vi "UHR-Fleezers Control (host) - 10.9.vi"() -> ()   [LabVIEW 2011] (continued)
        n1723 = local write "Set Reading to\nSetpoint"(FALSE ("Set SP to Reading")) -> ()
        n1724 = xnode "Read/Write Control"("FPGA VI Reference In"=w2622, "error in"=w2621) -> ("FPGA VI Reference Out"=w2620:T19, "error out"=w2619:errorcluster, "Trap Pos FB Int-Norm Signal"=w2618:fxp<+/-,16,1>)
        n1725 = local read "Differential FB?"() -> (w2623:bool)
        n1726 = case shown="False" w2623 {
          tunnel: [w2628 w2635] -> w2625
          tunnel: w2618 -> [w2626 w2635]
          frame False {
            n1727 = local read "Trap Pos FB Monitor\nT1 or T2"() -> (w2631:bool)
            n1728 = local read "Trap X AI1 (DMA)"() -> (w2634:T13)
            n1729 = Unbundle By Name(w2634) -> ("Set 1"=w2633:fxp<+/-,16,1>, "Set 2"=w2632:fxp<+/-,16,1>)
            n1730 = Select(t=w2633, s=w2631, f=w2632) -> (s? t:f=w2630:fxp<+/-,16,1>)
            n1731 = Not(x="Set SP Using...") -> (.not. x?=w2627:bool)
            n1732 = Select(t=w2626, s=w2627, f=w2630) -> (s? t:f=w2628:fxp<+/-,16,1>)
          }
          frame True {
          }
        }
        n1733 = xnode "Read/Write Control"("FPGA VI Reference In"=w2620, "error in"=w2619, "Trap Pos. FB SP"=w2625) -> ()  [unwired: 2 out]
        n1734 = local write "Trap Pos FB SP"(w2625) -> ()
      }
      event "Trap Pos. FB Out Scale 2^n": Value Change {
        n1735 = event-data() -> ()  [unwired: 7 out]
        n1736 = Scale By Power Of 2(n="Trap Pos. FB Out Scale 2^n", x=ext 1.0) -> (x*2^n=w2636:ext)
        n1737 = property on="Trap Pos. FB Mult Factor" class="DigNum (strict)"("Val(Sgnl)"=w2636) -> ()  [unwired: 2 in, 2 out]
      }
      event "Trap Pos FB Int Count": Value Change {
        n1738 = event-data() -> ()  [unwired: 7 out]
        n1739 = xnode "Read/Write Control"("FPGA VI Reference In"=w2641, "error in"=w2640, "Trap Pos FB Int Count"="Trap Pos FB Int Count") -> ()  [unwired: 2 out]
      }
    }
    "error out 2" <- w1554
    n1740 = node-c288() -> ()  [unwired: 2 out]
  }
  n1741 = timed-loop "Mouse control: trap position (AOM deflection), set confocal spot from image" {
    tunnel: [w2643] -> w182
    tunnel: w50 -> [w2642]
    timing: w94 -> [_]
    timing-out: [_] -> w93
    stop <- w2643 stop-if-true
    n1742 = node-c288() -> ()  [unwired: 2 out]
    n1743 = event shown="[0] \"Pane\": Mouse Down" {
      selector: _ -> [_ _]
      dyn-events: _ -> [_ _]
      timeout: _ -> [_ _]
      tunnel: w2642 -> [w2646 _]
      event Mouse Down {
        n1744 = event-data() -> ("Time"=w2648:u32, "Coords"=w2647:T7, "Button"=w2649:u16)  [unwired: 6 out]
        n1745 = case shown="1" w2649 {
          tunnel: w2648 -> [_ _ w2752]
          tunnel: w2647 -> [_ w2686 w2750]
          tunnel: w2646 -> [_ _ w2748]
          frame 0, Default {
          }
          frame 1 {
            n1746 = property on="APD 2" class="ImageControl"() -> ("Displayed Image Position"=w2656:cluster{"Left":i32, "Top":i32})  [unwired: 2 in, 2 out]
            n1747 = property on="APD 1" class="ImageControl"() -> ("Displayed Image Position"=w2685:cluster{"Left":i32, "Top":i32})  [unwired: 2 in, 2 out]
            n1748 = property on="Detection Laser X" class="ImageControl"() -> ("Displayed Image Position"=w2682:cluster{"Left":i32, "Top":i32})  [unwired: 2 in, 2 out]
            n1749 = property on="Detection Laser Y" class="ImageControl"() -> ("Displayed Image Position"=w2681:cluster{"Left":i32, "Top":i32})  [unwired: 2 in, 2 out]
            n1750 = property on="APD 2" class="ImageControl"() -> ("Displayed Image Size"=w2655:cluster{"Width":u32, "Height":u32})  [unwired: 2 in, 2 out]
            n1751 = property on="APD 1" class="ImageControl"() -> ("Displayed Image Size"=w2683:cluster{"Width":u32, "Height":u32})  [unwired: 2 in, 2 out]
            n1752 = property on="Detection Laser X" class="ImageControl"() -> ("Displayed Image Size"=w2684:cluster{"Width":u32, "Height":u32})  [unwired: 2 in, 2 out]
            n1753 = property on="Detection Laser Y" class="ImageControl"() -> ("Displayed Image Size"=w2680:cluster{"Width":u32, "Height":u32})  [unwired: 2 in, 2 out]
            n1754 = Unbundle By Name(w2655) -> ("Width"=w2652:u32, "Height"=w2651:u32)
            n1755 = Unbundle By Name(w2656) -> ("Left"=w2654:i32, "Top"=w2653:i32)
            n1756 = Unbundle By Name(w2683) -> ("Width"=w2677:u32, "Height"=w2676:u32)
            n1757 = Unbundle By Name(w2684) -> ("Width"=w2673:u32, "Height"=w2672:u32)
            n1758 = Unbundle By Name(w2680) -> ("Width"=w2669:u32, "Height"=w2668:u32)
            n1759 = Unbundle By Name(w2685) -> ("Left"=w2679:i32, "Top"=w2678:i32)
            n1760 = Unbundle By Name(w2682) -> ("Left"=w2675:i32, "Top"=w2674:i32)
            n1761 = Unbundle By Name(w2681) -> ("Left"=w2671:i32, "Top"=w2670:i32)
            n1762 = Bundle("Left"=w2654, "Top"=w2653, "Width"=w2652, "Height"=w2651) -> (w2650:T29)  [unwired: 1 in]
            n1763 = Bundle("Left"=w2679, "Top"=w2678, "Width"=w2677, "Height"=w2676) -> (w2667:T29)  [unwired: 1 in]
            n1764 = Bundle("Left"=w2675, "Top"=w2674, "Width"=w2673, "Height"=w2672) -> (w2666:T29)  [unwired: 1 in]
            n1765 = Bundle("Left"=w2671, "Top"=w2670, "Width"=w2669, "Height"=w2668) -> (w2665:T29)  [unwired: 1 in]
            n1766 = Build Cluster Array(w2650, w2667, w2666, w2665) -> (w2664:T30)
            n1767 = for {
              tunnel: w2686 -> [w2697]
              tunnel: w2664 -> [w2698] mode=indexing
              shift-right: [w2695] -> w2662
              shift-left: TRUE -> [w2696]
              shift-right: [w2694] -> w2660
              shift-left: _ -> [w2690]
              shift-right: [w2693] -> w2659
              shift-left: _ -> [w2689]
              shift-right: [w2692] -> w2658
              shift-left: _ -> [w2688]
              shift-right: [w2691] -> w2657
              shift-left: _ -> [w2687]
              n1768 = case shown="True" w2696 {
                selector: w2696 -> [w2703 _]
                tunnel: w2698 -> [_ w2712]
                tunnel: w2697 -> [_ w2710]
                tunnel: [w2703 w2708] -> w2695
                tunnel: [w2702 w2707] -> w2694
                tunnel: [w2701 w2706] -> w2693
                tunnel: [w2700 w2705] -> w2692
                tunnel: [w2699 w2704] -> w2691
                tunnel: w2690 -> [w2702 _]
                tunnel: w2689 -> [w2701 _]
                tunnel: w2688 -> [w2700 _]
                tunnel: w2687 -> [w2699 _]
                frame False {
                }
                frame True {
                  n1769 = Unbundle(w2712) -> (w2711:T29)
                  n1770 = call "isclickinwindow.vi"("Image Param"=w2711, "Point32"=w2710) -> ("4 Y"=w2704:i32, "3 Height"=w2705:i32, "2 X"=w2706:i32, "1 Width"=w2707:i32, "In image?"=w2709:bool)  [unwired: 1 in]
                  n1771 = Not(x=w2709) -> (.not. x?=w2708:bool)
                }
              }
            }
            n1772 = Not(x=w2662) -> (.not. x?=w2661:bool)
            n1773 = case shown="True" w2661 {
              tunnel: w2659 -> [_ w2725]
              tunnel: w2657 -> [_ w2724]
              tunnel: w2660 -> [_ w2723]
              tunnel: w2658 -> [_ w2722]
              frame False {
              }
              frame True {
                w2718 = FALSE ("Get Point")
                n1774 = local read "Scan lines (y)"() -> (w2727:u64)
                n1775 = local read "Actual MCL Inc (V)"() -> (w2719:dbl)
                n1776 = local read "Scan steps (MCL)"() -> (w2726:u64)
                n1777 = Divide "Y Pix/step"(x=w2722, y=w2727) -> (x/y=w2734:dbl)
                n1778 = Divide "Y V/pix"(x=w2719, y=w2734) -> (x/y=w2733:dbl)
                n1779 = Divide "Y half step offset"(x=w2719, y=2.0) -> (x/y=w2735:dbl)
                n1780 = Divide "X pix/step"(x=w2723, y=w2726) -> (x/y=w2732:dbl)
                n1781 = Negate(x=w2735) -> (-x=w2736:dbl)
                n1782 = local read "Initial Y"() -> (w2742:dbl)
                n1783 = Multiply(x=w2724, y=w2733) -> (x*y=w2743:dbl)
                n1784 = Divide "X half step offset"(x=w2719, y=2.0) -> (x/y=w2729:dbl)
                n1785 = Divide "X V/pix"(x=w2719, y=w2732) -> (x/y=w2731:dbl)
                n1786 = Multiply(x=w2719, y=w2726) -> (x*y=w2738:dbl)
                n1787 = Compound Arithmetic op=ADD(w2736, w2743, w2742) -> (w2720:dbl)
                "Pointer Y (V)" <- w2720
                n1788 = Multiply(x=w2731, y=w2725) -> (x*y=w2740:dbl)
                n1789 = Negate(x=w2729) -> (-x=w2728:dbl)
                n1790 = local read "Initial X"() -> (w2741:dbl)
                n1791 = Negate(x=w2740) -> (-x=w2739:dbl)
                n1792 = Compound Arithmetic op=ADD(w2728, w2738, w2741, w2739) -> (w2721:dbl)
                "Pointer X (V)" <- w2721
                n1793 = Or(x="Set X Only", y="Set Confocal Spot (X-Y)") -> (x .or. y?=w2714:bool)
                n1794 = Or(x="Set Confocal Spot (X-Y)", y="Set Y Only") -> (x .or. y?=w2713:bool)
                n1795 = case shown="True" w2714 {
                  tunnel: w2721 -> [_ w2744]
                  frame False {
                  }
                  frame True {
                    n1796 = property on="AO2" class="Slide (strict)"("Val(Sgnl)"=w2744) -> ()  [unwired: 2 in, 2 out]
                  }
                }
                n1797 = case shown="True" w2713 {
                  tunnel: w2720 -> [_ w2745]
                  frame False {
                  }
                  frame True {
                    n1798 = property on="AO1" class="Slide (strict)"("Val(Sgnl)"=w2745) -> ()  [unwired: 2 in, 2 out]
                  }
                }
                n1799 = local write "Set Confocal Spot (X-Y)"(w2718) -> ()
                n1800 = local write "Set X Only"(w2718) -> ()
                n1801 = local write "Set Y Only"(w2718) -> ()
              }
            }
          }
          frame 3 {
            n1802 = local read "BD 2 Frequency 1 (MHz)"() -> (w2746:dbl)
            n1803 = local read "BD 1 Frequency 1 (MHz)"() -> (w2747:dbl)
            n1804 = local write "Manipulating Trap"(TRUE ("Manipulating Trap")) -> ()
            n1805 = local write "Coords"(T7 {"Horizontal"=0, "Vertical"=0} ("Coords")) -> ()
            n1806 = while {
              tunnel: w2752 -> [w2757]
              tunnel: w2750 -> [w2756]
              tunnel: w2748 -> [w2755]
              tunnel: w2747 -> [w2754]
              tunnel: w2746 -> [w2753]
              stop <- w2758 stop-if-true
              n1807 = event shown="[0] \"Pane\": Mouse Move" {
                selector: _ -> [_ _]
                dyn-events: _ -> [_ _]
                timeout: _ -> [_ _]
                tunnel: ["Force Manip Abort" w2822] -> w2758
                tunnel: w2757 -> [w2765 _]
                tunnel: w2756 -> [w2763 _]
                tunnel: w2755 -> [w2762 _]
                tunnel: w2754 -> [w2761 _]
                tunnel: w2753 -> [w2760 _]
                event Mouse Move {
                  n1808 = event-data() -> ("Time"=w2766:u32, "Coords"=w2767:T7)  [unwired: 3 out]
                  n1809 = Less?(x=w2766, y=w2765) -> (x < y?=w2764:bool)
                  n1810 = case "Makes sure old motion events prior to mouse click aren't used" shown="False" w2764 {
                    tunnel: w2767 -> [w2809 _]
                    tunnel: w2763 -> [w2810 _]
                    tunnel: w2762 -> [w2787 _]
                    tunnel: w2761 -> [w2783 _]
                    tunnel: w2760 -> [w2782 _]
                    frame False {
                      n1811 = Subtract(x=w2809, y=w2810) -> (x-y=w2808:T7)
                      "Coords" <- w2808
                      n1812 = local read "Y RF Frequency Limits (MHz)"() -> (w2768:T16)
                      n1813 = To Double Precision Float(number=w2808) -> (double precision float=w2807:cluster{"Horizontal":dbl, "Vertical":dbl})
                      n1814 = Multiply(x=cluster{"Horizontal":dbl, "Vertical":dbl} {"Horizontal"=-1.0, "Vertical"=1.0}, y="Manipulation Scaling") -> (x*y=w2803:cluster{"Horizontal":dbl, "Vertical":dbl})
                      n1815 = local read "X RF Frequency Limits (MHz)"() -> (w2769:T16)
                      n1816 = Multiply(x=w2807, y=w2803) -> (x*y=w2805:cluster{"Horizontal":dbl, "Vertical":dbl})
                      n1817 = Unbundle By Name(w2805) -> ("Horizontal"=w2800:dbl, "Vertical"=w2804:dbl)
                      n1818 = Unbundle By Name(w2768) -> ("Maximum"=w2771:dbl, "Minimum"=w2770:dbl)
                      n1819 = Boolean To (0,1)(Boolean="Manip. X?") -> (0, 1=w2798:i16)
                      n1820 = Boolean To (0,1)(Boolean="Manip. Y?") -> (0, 1=w2795:i16)
                      n1821 = local read "BD 1 Frequency 2 (MHz)"() -> (w2785:dbl)
                      n1822 = Multiply(x=w2804, y=w2795) -> (x*y=w2797:dbl)
                      n1823 = Multiply(x=w2798, y=w2800) -> (x*y=w2801:dbl)
                      n1824 = local read "BD 2 Frequency 2 (MHz)"() -> (w2784:dbl)
                      n1825 = Unbundle By Name(w2769) -> ("Maximum"=w2773:dbl, "Minimum"=w2772:dbl)
                      n1826 = Add(x=w2782, y=w2797) -> (x+y=w2775:dbl)
                      n1827 = Add(x=w2783, y=w2801) -> (x+y=w2777:dbl)
                      n1828 = In Range and Coerce(upper limit=w2773, x=w2777, lower limit=w2772) -> (coerced(x)=w2776:dbl)  [unwired: 1 out]
                      n1829 = In Range and Coerce(upper limit=w2771, x=w2775, lower limit=w2770) -> (coerced(x)=w2774:dbl)  [unwired: 1 out]
                      n1830 = Subtract(x=w2776, y=w2785) -> (x-y=w2794:dbl)
                      n1831 = Subtract(x=w2774, y=w2784) -> (x-y=w2793:dbl)
                      n1832 = Square(x=w2794) -> (x^2=w2792:dbl)
                      n1833 = Square(x=w2793) -> (x^2=w2791:dbl)
                      n1834 = Add(x=w2792, y=w2791) -> (x+y=w2790:dbl)
                      n1835 = Square Root(x=w2790) -> (sqrt(x)=w2786:dbl)
                      n1836 = In Range and Coerce(upper limit="Limit Max (MHz)", x=w2786, lower limit="Limit Min (MHz)") -> (In Range?=w2779:bool)  [unwired: 1 out]
                      n1837 = Not(x="Limits Enable") -> (.not. x?=w2778:bool)
                      n1838 = Or(x=w2779, y=w2778) -> (x .or. y?=w2780:bool)
                      n1839 = case shown="True" w2780 {
                        tunnel: w2787 -> [_ w2820]
                        tunnel: w2786 -> [_ w2811]
                        tunnel: w2776 -> [_ w2818]
                        tunnel: w2785 -> [_ w2817]
                        tunnel: w2774 -> [_ w2816]
                        tunnel: w2784 -> [_ w2815]
                        tunnel: w2769 -> [_ w2813]
                        tunnel: w2768 -> [_ w2812]
                        frame False {
                        }
                        frame True {
                          n1840 = local read "BD 1 Frequency 3 (MHz)"() -> (w2819:dbl)
                          n1841 = local read "BD 2 Frequency 3 (MHz)"() -> (w2814:dbl)
                          n1842 = local write "Trap Delta (MHz)"(w2811) -> ()
                          n1843 = call "set RF board frequency - interlace.vi"("Board 2 Frequency Limits"=w2812, "Board 1 Frequency Limits"=w2813, "FPGA VI Reference In"=w2820, "Board 2 Frequency 3 (MHz)"=w2814, "Board 1 Frequency 3 (MHz)"=w2819, "Board 2 Frequency 2 (MHz)"=w2815, "Board 2 Frequency 1 (MHz)"=w2816, "Board 1 Frequency 2 (MHz)"=w2817, "Board 1 Frequency 1  (MHz)"=w2818) -> ()  [unwired: 1 in, 2 out]
                          n1844 = local write "BD 2 Frequency 1 (MHz)"(w2816) -> ()
                          n1845 = local write "BD 1 Frequency 1 (MHz)"(w2818) -> ()
                        }
                      }
                    }
                    frame True {
                    }
                  }
                }
                event Mouse Up {
                  n1846 = event-data() -> ("Button"=w2821:u16)  [unwired: 8 out]
                  n1847 = case shown="3" w2821 {
                    tunnel: [FALSE TRUE] -> w2822
                    frame 0, Default {
                    }
                    frame 3 {
                      n1848 = local read "Trap Delta (MHz)"() -> (w2824:dbl)
                      n1849 = property on="Initial delta (MHz)" class="DigNum (strict)"("Val(Sgnl)"=w2824) -> ()  [unwired: 2 in, 2 out]
                      n1850 = local write "Manipulating Trap"(FALSE ("Manipulating Trap")) -> ()
                    }
                  }
                }
              }
            }
          }
        }
      }
      event Mouse Move {
        n1851 = event-data() -> ()  [unwired: 6 out]
      }
    }
    n1852 = local read "Stop All"() -> (w2643:bool)
    n1853 = node-c288() -> ()  [unwired: 2 out]
  }
  n1854 = node-c288(w91) -> ()  [unwired: 1 out]
  n1855 = node-c288(w93) -> ()  [unwired: 1 out]
  n1856 = flat-sequence "Video" {
    tunnel: [w2835] -> w80
    tunnel: w80 -> [w2876]
    frame #0 {
      n1857 = while {
        stop <- w2828 continue-if-true
        n1858 = call "Close Video Capture.vi"() -> ("error code OUT"=w2830:i32)
        n1859 = Equal?(x=w2830, y=0) -> (x = y?=w2828:bool)
      }
      n1860 = local write "Stop All"(FALSE ("Stop All")) -> ()
    }
    frame #1 {
      n1861 = call "DMR_Init.vi"() -> ()  [unwired: 3 out]
    }
    frame #2 {
      # "Setting the destination format to Mono8 makes sure that the image can be displayed in the intensity plot."
      n1862 = call "DMR_GetDevice.vi"("search string IN"="DE019116701") -> ("device handle OUT"=w2853:i32)  [unwired: 4 in, 2 out]
      n1863 = call "DMR_OpenDevice.vi"("device handle IN"=w2853) -> ("driver handle OUT"=w2836:i32)  [unwired: 4 out]
      n1864 = call "DMR_FindList.vi"("flags IN"=u32 0 ("flags"), "list name IN"="" ("String"), "list type IN"=T31."camera descriptions", "driver handle IN"=w2836) -> ("list handle OUT"=w2839:i32)  [unwired: 2 out]
      n1865 = call "DMR_FindList.vi"("flags IN"=u32 0 ("flags"), "list name IN"="Base", "list type IN"=T31."setting", "driver handle IN"=w2836) -> ("list handle OUT"=w2837:i32)  [unwired: 2 out]
      n1866 = call "OBJ_GetHandle.vi"("object name IN"="VideoStandard", "list handle IN"=w2839) -> ("object handle OUT"=w2833:i32)  [unwired: 3 out]
      n1867 = call "OBJ_GetHandle.vi"("object name IN"="PixelFormat", "list handle IN"=w2837) -> ("object handle OUT"=w2847:i32)  [unwired: 3 out]
      n1868 = call "OBJ_SetS.vi"("value index IN"=0, "value IN"="NTSC M", "object handle IN"=w2833) -> ()  [unwired: 2 out]
      n1869 = call "OBJ_SetS.vi"("value index IN"=0, "value IN"="Mono8" ("value"), "object handle IN"=w2847) -> ()  [unwired: 2 out]
      n1870 = call "OBJ_GetHandle.vi"("object name IN"="VideoChannel", "list handle IN"=w2837) -> ("object handle OUT"=w2843:i32)  [unwired: 3 out]
      n1871 = while {
        tunnel: [w2858] -> w2835
        tunnel: w2836 -> [w2855]
        stop <- w2856 continue-if-true
        n1872 = call "DMR_ImageRequestSingle.vi"("request control IN"=0, "driver handle IN"=w2855) -> ("error code OUT"=w2857:i32, "driver handle OUT"=w2858:i32)  [unwired: 2 out]
        n1873 = Equal To 0?(x=w2857) -> (x = 0?=w2856:bool)
      }
      n1874 = call "OBJ_SetI.vi"("value index IN"=0, "value IN"=3 ("Video channel"), "object handle IN"=w2843) -> ()  [unwired: 2 out]
    }
    frame #3 {
      w2864 = T17 0 items=["Grayscale (U8)", "Grayscale (I16)", "Grayscale (SGL)", "Complex (CSG)", "RGB (U32)", "HSL (U32)", "RGB (U64)"] ("Image Type")
      w2872 = T17 0 items=["Grayscale (U8)", "Grayscale (I16)", "Grayscale (SGL)", "Complex (CSG)", "RGB (U32)", "HSL (U32)", "RGB (U64)"] ("Image Type")
      n1875 = for "Create Greyscale map" {
        N: 256 -> [_]
        tunnel: [w2878] -> w2861 mode=indexing
        workers-P: _ -> [_]
        i -> [w2881]
        n1876 = To Unsigned Byte Integer(number=w2881) -> (unsigned 8bit integer=w2877:u8)
        n1877 = Join Numbers(hi=w2877, lo=w2877) -> ((hi.lo)=w2880:u16)
        n1878 = Join Numbers(hi=w2877, lo=w2877) -> ((hi.lo)=w2879:u16)
        n1879 = Join Numbers(hi=w2880, lo=w2879) -> ((hi.lo)=w2878:u32)
      }
      n1880 = call "IMAQ Create"("Image Name"="Scaled video", "Image Type"=w2864) -> ("New Image"=w2863:T2)  [unwired: 2 in, 2 out]
      n1881 = call "IMAQ Create"("Image Name"="Main video", "Image Type"=w2872) -> ("New Image"=w2873:T2)  [unwired: 2 in, 2 out]
      n1882 = node-c288(0 ("Processor")) -> (w2871:T21)  [unwired: 3 out]
      n1883 = Initialize Array(u32 0 ("Window Number (0...15)"), 480 ("dimension size"), 640 ("dimension size")) -> (w2866:u32[][])
      n1884 = timed-loop {
        tunnel: w2876 -> [w2898]
        tunnel: [w2897] -> w2875
        tunnel: w2873 -> [w2896]
        timing: w2871 -> [_]
        timing-out: [_] -> w2870
        tunnel: w2866 -> [w2885]
        tunnel: w2863 -> [w2883]
        tunnel: w2861 -> [w2882]
        stop <- w2884 stop-if-true
        # "This block performs the \nactual image capture."
        n1885 = node-c288() -> ()  [unwired: 2 out]
        n1886 = local read "Stop All"() -> (w2884:bool)
        n1887 = Reciprocal(x="Video Capture Rate (Hz)") -> (1/x=w2888:dbl)
        n1888 = Multiply(x=w2888, y=1000.0) -> (x*y=w2886:dbl)
        n1889 = call "DMR_ImageRequestWaitFor.vi"("queue number IN"=0, "timeout(ms) IN"=500, "driver handle IN"=w2898) -> ("error code OUT"=w2902:i32, "request number OUT"=w2899:i32, "driver handle OUT"=w2900:i32)
        n1890 = feedback #1(T32 refnum ("Avi Refnum")) -> (w2890:T32)
        n1891 = case shown="True" "New Video File" {
          tunnel: [T32 refnum ("Avi Refnum") w2919] -> w2892
          tunnel: [FALSE TRUE] -> w2893
          tunnel: w2890 -> [_ w2915]
          frame False {
          }
          frame True {
            n1892 = call "Create new save file.vi"("Ext"=".avi" ("string"), "Index In"="Video Index") -> ("Path Out"=w2911:path, "Index Out"=w2912:dbl)  [unwired: 1 in]
            "Path Out" <- w2911
            n1893 = Not Equal?(x=w2915, y=T32 refnum ("Avi Refnum")) -> (x != y?=w2916:bool)
            n1894 = Increment(x=w2912) -> (x+1=w2921:dbl)
            n1895 = case shown="True" w2916 {
              tunnel: w2915 -> [_ w2922]
              frame False {
              }
              frame True {
                n1896 = call "IMAQ AVI Close"("Avi Refnum"=w2922) -> ()  [unwired: 1 in, 10 out]
              }
            }
            n1897 = local write "Video Index"(w2921) -> ()
            n1898 = call "IMAQ AVI Create"("Frames Per Second"=u32 30, "AVI Path"=w2911) -> ("Avi Refnum"=w2919:T32)  [unwired: 5 in, 4 out]
          }
        }
        n1899 = Equal To 0?(x=w2902) -> (x = 0?=w2901:bool)
        n1900 = Select(t=w2892, s=w2893, f=w2890) -> (s? t:f=w2891:T32)
        n1901 = feedback-in #1(w2891) -> ()
        n1902 = case shown="True" w2901 {
          tunnel: w2900 -> [w2923 w2948]
          tunnel: w2899 -> [_ w2947]
          tunnel: [w2923 w2944] -> w2897
          tunnel: w2896 -> [_ w2928]
          tunnel: w2885 -> [_ w2932]
          tunnel: w2891 -> [_ w2930]
          tunnel: w2883 -> [_ w2925]
          tunnel: w2882 -> [_ w2924]
          frame False {
          }
          frame True {
            w2938 = u32 0 ("X-offset IN")
            n1903 = call "DMR_GetImageRequestBufferData.vi"("driver handle IN"=w2948, "request number IN"=w2947) -> ("width OUT"=w2937:i32, "height OUT"=w2936:i32, "driver handle OUT"=w2943:i32, "request number OUT"=w2942:i32, "bytes per pixel OUT"=w2939:i32)  [unwired: 13 out]
            n1904 = call "DMR_GetImageRequestBufferImageData.vi"("driver handle IN"=w2943, "request number IN"=w2942, "bytes per pixel IN"=w2939, "X-offset IN"=w2938, "Y-offset IN"=w2938, "height IN"=w2936, "width IN"=w2937) -> ("driver handle OUT"=w2941:u32, "request number OUT"=w2940:u32, "image OUT"=w2933:u32[][])  [unwired: 10 out]
            n1905 = call "DMR_ImageRequestUnlock.vi"("request number IN"=w2940, "driver handle IN"=w2941) -> ("driver handle OUT"=w2946:i32)  [unwired: 1 in, 2 out]
            n1906 = case shown="True" "Averaging" {
              tunnel: w2933 -> [w2984 w2989]
              tunnel: [w2984 w2988] -> w2929
              tunnel: w2932 -> [_ w2986]
              frame False {
              }
              frame True {
                (unwired) 1
                w2994 = 1
                n1907 = feedback #2(w2986) -> (w2985:u32[][])
                n1908 = Add(x=w2989, y=w2985) -> (x+y=w2990:u32[][])
                n1909 = Select(t=w2986, s="Reset Averaging", f=w2990) -> (s? t:f=w2992:u32[][])
                n1910 = feedback-in #2(w2992) -> ()
                n1911 = feedback #3(w2994) -> (w2987:i32)
                n1912 = Divide(x=w2990, y=w2987) -> (x/y=w2991:dbl[][])
                n1913 = Increment(x=w2987) -> (x+1=w2995:i32)
                n1914 = To Unsigned Long Integer(number=w2991) -> (unsigned 32bit integer=w2988:u32[][])
                n1915 = Select(t=w2994, s="Reset Averaging", f=w2995) -> (s? t:f=w2993:i32)
                n1916 = feedback-in #3(w2993) -> ()
              }
            }
            n1917 = call "DMR_ImageRequestSingle.vi"("request control IN"=0, "driver handle IN"=w2946) -> ("driver handle OUT"=w2944:i32)  [unwired: 3 out]
            n1918 = disable-structure shown="Disabled" {
              disable-tunnel: w2929 -> [w2961 _]
              disable-tunnel: w2925 -> [w2960 _]
              frame Disabled {
                n1919 = To Double Precision Float(number=w2961) -> (double precision float=w2959:dbl[][])
                n1920 = In Range and Coerce(upper limit="Intensity Upper", x=w2959, lower limit="Intensity Lower") -> (coerced(x)=w2958:dbl[][])  [unwired: 1 out]
                n1921 = Subtract(x="Intensity Upper", y="Intensity Lower") -> (x-y=w2955:dbl)
                n1922 = Subtract(x=w2958, y="Intensity Lower") -> (x-y=w2956:dbl[][])
                n1923 = Divide(x=w2956, y=w2955) -> (x/y=w2957:dbl[][])
                n1924 = Multiply(x=255.0, y=w2957) -> (x*y=w2953:dbl[][])
                n1925 = To Unsigned Byte Integer(number=w2953) -> (unsigned 8bit integer=w2962:u8[][])
                n1926 = call "IMAQ ArrayToImage"("Image Pixels (U8)"=w2962, "Image"=w2960) -> ("Image Out"=w2949:T2)  [unwired: 4 in, 5 out]
                n1927 = First Call?() -> (First Call?: T/F=w2950:bool)
                n1928 = case shown="True" w2950 {
                  tunnel: w2949 -> [w2963 w2974]
                  frame False {
                    n1929 = flat-sequence {
                      tunnel: w2963 -> [w2969]
                      frame #0 {
                        w2966 = FALSE ("Get/Set Status? (Set)")
                        w2965 = 0 ("Window Number (0...15)")
                        n1930 = call "IMAQ WindSize"("Get/Set Status? (Set)"=w2966, "Window Number"=w2965) -> ("Width & Height out"=→"Window Size":cluster{"Width":i32, "Height":i32})  [unwired: 4 in, 2 out]
                        n1931 = call "IMAQ WindMove"("Window Number (0...15)"=w2965, "Get/Set Status? (Set)"=w2966) -> ("Coordinates (screen)"=→"Window Position":cluster{"X Position":i32, "Y Position":i32})  [unwired: 3 in, 1 out]
                        n1932 = call "IMAQ WindDraw"("Resize to Image Size? (Y)"=FALSE, "Window Number (0...15)"=w2965, "Image"=w2969) -> ()  [unwired: 7 in, 2 out]
                      }
                      frame #1 {
                        n1933 = call "IMAQ WindZoom 2"("Center Point"="Center Point", "Zoom to Fit? (False)"=FALSE, "Zoom Factor"="Zoom Factor") -> ()  [unwired: 5 in, 4 out]
                      }
                    }
                  }
                  frame True {
                    n1934 = flat-sequence {
                      tunnel: w2974 -> [w2977]
                      tunnel: [w2975] -> w2973
                      tunnel: w2973 -> [w2979]
                      frame #0 {
                        w2976 = TRUE ("Resize to Image Size? (Y)")
                        w2975 = 0 ("Window Number (0...15)")
                        n1935 = call "IMAQ WindNonTearing"("Window Number"=w2975, "NonTearing? (True)"=w2976) -> ()  [unwired: 8 in, 2 out]
                        n1936 = call "IMAQ WindDraw"("Resize to Image Size? (Y)"=w2976, "Window Number (0...15)"=w2975, "Image"=w2977) -> ()  [unwired: 7 in, 2 out]
                      }
                      frame #1 {
                        n1937 = call "IMAQ WindSize"("Scrollbars? (N)"=FALSE, "Width & Height"="Initial Window Size", "Window Number"=w2979) -> ()  [unwired: 3 in, 3 out]
                        n1938 = call "IMAQ WindMove"("Window Number (0...15)"=w2979, "Coordinates (screen)"="Initial Window Position") -> ()  [unwired: 3 in, 2 out]
                      }
                    }
                  }
                }
              }
              frame Enabled {
              }
            }
            n1939 = To Unsigned Byte Integer(number=w2929) -> (unsigned 8bit integer=w2927:u8[][])
            n1940 = call "IMAQ ArrayToImage"("Image Pixels (U8)"=w2927, "Image"=w2928) -> ("Image Out"=w2926:T2)  [unwired: 4 in, 5 out]
            "Primary Video Display" <- w2926
            n1941 = case shown="True" "Save Video" {
              tunnel: w2930 -> [_ w2983]
              tunnel: w2926 -> [_ w2982]
              frame False {
              }
              frame True {
                n1942 = call "IMAQ AVI Write Frame"("Image"=w2982, "Avi Refnum"=w2983) -> ()  [unwired: 2 in, 8 out]
              }
            }
            n1943 = case shown="True" "Save Image" {
              tunnel: w2927 -> [_ w2998]
              tunnel: w2924 -> [_ w2997]
              frame False {
              }
              frame True {
                n1944 = call <vilib>:"Flatten Pixmap.vi"("colors"=w2997, "8-bit pixmap"=w2998) -> ("image data"=w3004:T33)  [unwired: 4 in, 5 out]
                n1945 = call "Create new save file.vi"("Insert"="video_frame_" ("string"), "Ext"=".bmp" ("string"), "Index In"="Image Index") -> ("Path Out"=w3000:path, "Index Out"=w3005:dbl)
                n1946 = Increment(x=w3005) -> (x+1=w2999:dbl)
                n1947 = local write "Image Index"(w2999) -> ()
                n1948 = call <vilib>:"Write BMP File.vi"("image data"=w3004, "path to BMP file"=w3000) -> ()  [unwired: 1 in, 9 out]
              }
            }
          }
        }
        n1949 = node-c288(w2886) -> ()  [unwired: 1 out]
      }
      n1950 = node-c288(w2870) -> ()  [unwired: 1 out]
      n1951 = call "DMR_CloseDevice.vi"("driver handle IN"=w2875) -> ()  [unwired: 1 in, 4 out]
    }
    frame #4 {
      n1952 = call "DMR_Close.vi"() -> ()  [unwired: 1 out]
    }
  }
  n1953 = node-c288(i64 1 ("Period"), 1 ("Processor")) -> (w175:T21)  [unwired: 2 out]
  n1954 = timed-loop "Acquire Data" {
    tunnel: w50 -> [w3304]
    tunnel: w49 -> [w3303]
    tunnel: [w3333] -> w270
    tunnel: [w3328] -> w268
    timing: w175 -> [_]
    timing-out: [_] -> w174
    tunnel: w69 -> [w3141]
    stop <- "Stop All" stop-if-true
    w3056 = "Initialize"
    w3126 = "NI_ChannelName" ("name")
    n1955 = node-c288() -> ()  [unwired: 2 out]
    n1956 = First Call?() -> (First Call?: T/F=w3091:bool)
    n1957 = Or(x="Reset", y=w3091) -> (x .or. y?=w3092:bool)
    n1958 = local read "Flushing P1"() -> (w3010:bool)
    n1959 = case "Reset data stream" shown="True" w3092 {
      tunnel: w3304 -> [w4309 w4317]
      tunnel: w3303 -> [w4308 w4316]
      tunnel: [w4309 w4311] -> w3299
      tunnel: [w4308 w4310] -> w3298
      frame False {
      }
      frame True {
        w4314 = TRUE ("AI to FIFO")
        n1960 = local write "Overflow (data lost)"(FALSE ("Overflow (data lost)")) -> ()
        n1961 = call "reset FPGA DMA.vi"("error in"=w4316, "FPGA VI Reference In"=w4317) -> ("error out"=w4312:errorcluster, "FPGA VI Reference Out"=w4313:T19)
        n1962 = xnode "Read/Write Control"("FPGA VI Reference In"=w4313, "error in"=w4312, "AI to FIFO"=w4314, "APD to FIFO"=w4314) -> ("FPGA VI Reference Out"=w4311:T19, "error out"=w4310:errorcluster)
      }
    }
    n1963 = case shown="True" w3010 {
      frame False {
      }
      frame True {
        n1964 = local read "Flush rate (uL/m) P1"() -> (w3350:dbl)
        n1965 = local read "HP1 Flush Time (s)"() -> (w3359:dbl)
        n1966 = local read "DMA Update Period (s)"() -> (w3353:dbl)
        n1967 = Divide(x=w3350, y=60.0) -> (x/y=w3351:dbl)
        n1968 = Divide(x=w3359, y=w3353) -> (x/y=w3348:dbl)
        n1969 = feedback #4(0) -> (w3357:i32)
        n1970 = Increment(x=w3357) -> (x+1=w3347:i32)
        n1971 = Greater?(x=w3347, y=w3348) -> (0:w3356:bool)
        n1972 = Compound Arithmetic op=MULTIPLY(w3353, w3347, w3351) -> (→"P1 Flush Volume (uL)":dbl)
        n1973 = Divide(x=w3347, y=w3348) -> (x/y=→"P1 Flushing Bar":dbl)
        n1974 = case shown="True" w3356 {
          tunnel: w3347 -> [w3360 _]
          tunnel: [w3360 0] -> w3355
          frame False {
          }
          frame True {
            w3361 = FALSE ("Flushing P1")
            n1975 = local write "Inject Pump 1"(w3361) -> ()
            n1976 = local write "Flushing P1"(w3361) -> ()
            n1977 = property on="Clear Volume P1" class="Bool (strict)"("Val(Sgnl)"=TRUE ("Value (Signaling)")) -> ()  [unwired: 2 in, 2 out]
          }
        }
        n1978 = feedback-in #4(w3355) -> ()
      }
    }
    n1979 = Or(x="Start AOD Scan", y="Trap Raster Scan") -> (x .or. y?=w3249:bool)
    n1980 = case "Start AOM raster scan" shown="True" w3249 {
      tunnel: w3299 -> [w4159 w4169]
      tunnel: w3298 -> [w4158 w4168]
      tunnel: [w4159 w4162] -> w3297
      tunnel: [w4158 w4161] -> w3296
      frame False {
      }
      frame True {
        n1981 = case shown="True" "Restart DMA? (AOD)" {
          tunnel: [w4207 w4209] -> w4163
          tunnel: [w4206 w4208] -> w4164
          tunnel: w4169 -> [w4207 w4211]
          tunnel: w4168 -> [w4206 w4210]
          frame False {
          }
          frame True {
            n1982 = local write "Overflow (data lost)"(FALSE ("Overflow (data lost)")) -> ()
            n1983 = call "reset FPGA DMA.vi"("error in"=w4210, "FPGA VI Reference In"=w4211) -> ("error out"=w4208:errorcluster, "FPGA VI Reference Out"=w4209:T19)
          }
        }
        n1984 = local write "Trap Raster Scan"(FALSE ("Trap Raster Scan")) -> ()
        n1985 = case shown="True" "Move MCL Also?" {
          tunnel: w4164 -> [w4172 w4201]
          tunnel: w4163 -> [w4173 w4202]
          tunnel: [w4171 w4205] -> w4162
          tunnel: [w4170 w4204] -> w4161
          frame False {
            w4174 = TRUE ("AI to FIFO")
            n1986 = xnode "Read/Write Control"("FPGA VI Reference In"=w4173, "error in"=w4172, "AI to FIFO"=w4174, "APD to FIFO"=w4174, "Start scan"=w4174) -> ("FPGA VI Reference Out"=w4171:T19, "error out"=w4170:errorcluster)
          }
          frame True {
            w4198 = FALSE ("1D or 2D Scan?")
            w4203 = TRUE ("AI to FIFO")
            # "Count for MCL loop"
            # "N total cycles"
            # "N steps"
            # "V_int"
            n1987 = local read "Scan Range (nm)"() -> (w4180:dbl)
            n1988 = local read "Number of F/B Scans (AOD)"() -> (w4197:u16)
            n1989 = Sign(1:w4180) -> (0:w4179:dbl)
            n1990 = Compound Arithmetic op=MULTIPLY(w4180, "MCL Step Position Ratio", "MCL/AOM Scale Tweak") -> (w4184:dbl)
            n1991 = Negate(x=w4179) -> (-x=w4176:dbl)
            n1992 = Multiply(x=w4176, y="MCL Step Increment (V_int)") -> (x*y=w4178:dbl)
            n1993 = Divide(x=w4184, y="MCL X Cal (nm/V)") -> (x/y=w4190:dbl)
            n1994 = Multiply(x=32767.0 ("y"), y=w4190) -> (x*y=w4196:dbl)
            n1995 = local read "Total Counts (ticks)"() -> (w4181:u32)
            n1996 = local read "Cycles/step (AOD)"() -> (w4192:u64)
            n1997 = local read "Scan steps (AOD)"() -> (w4193:u64)
            n1998 = Divide(x=w4196, y=10.0) -> (x/y=w4189:dbl)
            n1999 = Divide(x=w4189, y="MCL Step Increment (V_int)") -> (x/y=w4187:dbl)
            n2000 = Absolute Value(x=w4187) -> (abs(x)=w4175:dbl)
            n2001 = Compound Arithmetic op=MULTIPLY(w4193, w4192, w4181) -> (w4188:u64)
            n2002 = local write "wait to reset values"(w4203) -> ()
            n2003 = local write "MCL Scanning"(w4203) -> ()
            n2004 = Divide(x=w4188, y=w4175) -> (x/y=w4185:dbl)
            "MCL Count" <- w4185
            n2005 = xnode "Read/Write Control"("FPGA VI Reference In"=w4202, "error in"=w4201, "Scan steps (MCL)"=w4175, "Number of scans (MCL)"=w4197, "Cycles per step (MCL)"=u64 1, "Scan freq.  increment (MCL)"=w4178, "1D or 2D Scan?"=w4198, "MCL Scan Axis"=w4198, "Cont. Scan (MCL)"=w4198, "MCL count"=w4185) -> ("FPGA VI Reference Out"=w4200:T19, "error out"=w4199:errorcluster)
            n2006 = xnode "Read/Write Control"("FPGA VI Reference In"=w4200, "error in"=w4199, "AI to FIFO"=w4203, "APD to FIFO"=w4203, "Start scan"=w4203, "Start scan (MCL)"=w4203) -> ("FPGA VI Reference Out"=w4205:T19, "error out"=w4204:errorcluster)
          }
        }
        "Raster Scanning..." <- TRUE ("Scanning...")
      }
    }
    n2007 = local read "Flushing P3"() -> (w3011:bool)
    n2008 = case "Keep track of when Harvard Pump 3 is done flushing" shown="True" w3011 {
      frame False {
      }
      frame True {
        n2009 = local read "Flush rate (uL/m) P3"() -> (w3367:dbl)
        n2010 = local read "DMA Update Period (s)"() -> (w3369:dbl)
        n2011 = local read "HP3 Flush Time (s)"() -> (w3376:dbl)
        n2012 = Divide(x=w3367, y=60.0) -> (x/y=w3365:dbl)
        n2013 = feedback #5(0) -> (w3374:i32)
        n2014 = Increment(x=w3374) -> (x+1=w3368:i32)
        n2015 = Divide(x=w3376, y=w3369) -> (x/y=w3370:dbl)
        n2016 = Greater?(x=w3368, y=w3370) -> (0:w3373:bool)
        n2017 = Compound Arithmetic op=MULTIPLY(w3369, w3368, w3365) -> (→"P3 Flush Volume (uL)":dbl)
        n2018 = case shown="True" w3373 {
          tunnel: w3368 -> [w3377 _]
          tunnel: [w3377 0] -> w3372
          frame False {
          }
          frame True {
            w3378 = FALSE ("Flushing P3")
            n2019 = local write "Inject Pump 3"(w3378) -> ()
            n2020 = local write "Flushing P3"(w3378) -> ()
            n2021 = property on="Clear Volume P3" class="Bool (strict)"("Val(Sgnl)"=TRUE ("Value (Signaling)")) -> ()  [unwired: 2 in, 2 out]
          }
        }
        n2022 = feedback-in #5(w3372) -> ()
        n2023 = Divide(x=w3368, y=w3370) -> (x/y=→"P3 Flushing Bar":dbl)
      }
    }
    n2024 = And(x="Save scans", y=w3249) -> (x .and. y?=w3295:bool)
    n2025 = Compound Arithmetic op=OR("Start MCL Scan", "Confocal Image", "Confocal Linescan") -> (w3247:bool)
    n2026 = And(x="Save Data (MCL)", y=w3247) -> (x .and. y?=w3294:bool)
    n2027 = case "Start MCL raster scan" shown="True" w3247 {
      tunnel: w3297 -> [w3776 w3792]
      tunnel: w3296 -> [w3775 w3791]
      tunnel: [w3776 w3787] -> w3139
      tunnel: [w3775 w3786] -> w3138
      tunnel: [FALSE w3785] -> w3280
      tunnel: "Start MCL Scan" -> [_ w3780]
      tunnel: "Confocal Image" -> [_ w3779]
      tunnel: "Confocal Linescan" -> [_ _]
      frame False {
      }
      frame True {
        w3785 = TRUE
        n2028 = case shown="True" "Restart DMA? (MCL)" {
          tunnel: [w3837 w3839] -> w3790
          tunnel: [w3836 w3838] -> w3789
          tunnel: w3792 -> [w3837 w3842]
          tunnel: w3791 -> [w3836 w3841]
          frame False {
          }
          frame True {
            n2029 = call "reset FPGA DMA.vi"("error in"=w3841, "FPGA VI Reference In"=w3842) -> ("error out"=w3838:errorcluster, "FPGA VI Reference Out"=w3839:T19)
            n2030 = local write "Overflow (data lost)"(FALSE ("Overflow (data lost)")) -> ()
          }
        }
        n2031 = case shown="False" w3780 {
          selector: w3780 -> [_ w3796]
          tunnel: w3779 -> [w3795 _]
          tunnel: [w3795 w3796] -> w3778
          frame False {
            n2032 = property on="2D or 1D Scan" class="Bool (strict)"("Val(Sgnl)"=w3795) -> ()  [unwired: 2 in, 2 out]
            n2033 = property on="Confocal Image" class="Bool (strict)"("Value"=FALSE ("Start Confocal Map")) -> ()  [unwired: 2 in, 2 out]
          }
          frame True {
          }
        }
        n2034 = local write "MCL Scanning"(w3785) -> ()
        n2035 = local read "AO1"() -> (w3782:dbl)
        n2036 = local read "AO2"() -> (w3781:dbl)
        n2037 = case shown="True" "Center Scan" {
          tunnel: w3790 -> [w3803 w3835]
          tunnel: w3789 -> [w3802 w3834]
          tunnel: [w3801 w3833] -> w3787
          tunnel: [w3800 w3832] -> w3786
          tunnel: [w3798 w3819] -> w3784
          tunnel: [w3797 w3818] -> w3783
          tunnel: w3782 -> [w3798 w3824]
          tunnel: w3781 -> [w3797 w3827]
          tunnel: w3778 -> [_ _]
          frame False {
            w3799 = TRUE ("AI to FIFO")
            n2038 = xnode "Read/Write Control"("FPGA VI Reference In"=w3803, "error in"=w3802, "AI to FIFO"=w3799, "APD to FIFO"=w3799, "Start scan (MCL)"=w3799) -> ("FPGA VI Reference Out"=w3801:T19, "error out"=w3800:errorcluster)
          }
          frame True {
            w3831 = TRUE ("AI to FIFO")
            n2039 = local read "Scan steps (MCL)"() -> (w3810:u64)
            n2040 = local read "Scan lines (y)"() -> (w3806:u64)
            n2041 = local read "Fast Scan Dir"() -> (w3817:bool)
            n2042 = local read "Actual MCL Inc (V)"() -> (w3807:dbl)
            n2043 = Decrement(x=w3806) -> (x-1=w3805:u64)
            n2044 = Decrement(x=w3810) -> (x-1=w3809:u64)
            n2045 = Multiply(x=w3807, y=w3805) -> (x*y=w3804:dbl)
            n2046 = Divide(x=w3804, y=2.0) -> (x/y=w3814:dbl)
            n2047 = Multiply(x=w3807, y=w3809) -> (x*y=w3808:dbl)
            n2048 = Divide(x=w3808, y=2.0) -> (x/y=w3813:dbl)
            n2049 = Select(t=w3813, s=w3817, f=w3814) -> (s? t:f=w3812:dbl)
            n2050 = Select(t=w3814, s=w3817, f=w3813) -> (s? t:f=w3816:dbl)
            n2051 = Subtract(x=w3824, y=w3816) -> (x-y=w3815:dbl)
            n2052 = Subtract(x=w3827, y=w3812) -> (x-y=w3811:dbl)
            n2053 = local read "2D or 1D Scan"() -> (w3829:bool)
            n2054 = Not(x=w3817) -> (.not. x?=w3823:bool)
            n2055 = Not(x=w3829) -> (.not. x?=w3825:bool)
            n2056 = And(x=w3817, y=w3825) -> (x .and. y?=w3826:bool)
            n2057 = And(x=w3825, y=w3823) -> (x .and. y?=w3828:bool)
            n2058 = Select(t=w3827, s=w3828, f=w3811) -> (s? t:f=w3818:dbl)
            n2059 = Select(t=w3824, s=w3826, f=w3815) -> (s? t:f=w3819:dbl)
            n2060 = call "Volt to I16.vi"("Voltage In"=w3819) -> ("I16 Voltage Out"=w3822:i16)
            n2061 = call "Volt to I16.vi"("Voltage In"=w3818) -> ("I16 Voltage Out"=w3821:i16)
            n2062 = xnode "Read/Write Control"("FPGA VI Reference In"=w3835, "error in"=w3834, "AI to FIFO"=w3831, "APD to FIFO"=w3831, "Start scan (MCL)"=w3831, "AO1"=w3822, "AO2"=w3821) -> ("FPGA VI Reference Out"=w3833:T19, "error out"=w3832:errorcluster)
          }
        }
        "Initial Y" <- w3784
        "Initial X" <- w3783
        n2063 = local write "Tab Control 6"(T3."Imaging" ("Tab Control 6")) -> ()
        "wait to reset values" <- w3785
      }
    }
    n2064 = local read "Trap Pos Elements/DMA read"() -> (w3135:u32)
    n2065 = local read "Trap AI Elements/DMA read"() -> (w3210:u32)
    n2066 = local read "APD Elements/DMA read"() -> (w3176:u32)
    n2067 = xnode "Get APD Data"("FPGA VI Reference In"=w3139, "error in"=w3138, "Number of Elements"=w3176, "Timeout (ms)"=-1) -> ("Data"=w3175:u32[], "Elements Remaining"=→"APD FIFO Elements Remaining":u32)  [unwired: 2 out]
    n2068 = xnode "Invoke Method"("FPGA VI Reference In"=w3139, "error in"=w3138, "Number of Elements"=w3135, "Timeout (ms)"=-1) -> ("Data"=w3098:u16[], "Elements Remaining"=→"Trap Pos FIFO El Remaining":u32)  [unwired: 2 out]
    n2069 = xnode "Get Trap Data"("FPGA VI Reference In"=w3139, "error in"=w3138, "Number of Elements"=w3210, "Timeout (ms)"=-1 ("Timeout")) -> ("FPGA VI Reference Out"=w3032:T19, "error out"=w3031:errorcluster, "Data"=w3099:i16[], "Elements Remaining"=w3341:u32)
    "FIFO El. Rem." <- w3341
    n2070 = local read "Trap AI FIFO Depth"() -> (w3343:u32)
    n2071 = Subtract(x=w3343, y=w3210) -> (x-y=w3342:u32)
    n2072 = Decimate 1D Array(w3098) -> (w3095:u16[], w3097:u16[], w3096:u16[])
    n2073 = Divide(x=w3341, y=w3342) -> (x/y=w3340:dbl)
    "Buffer Status" <- w3340
    n2074 = To Unsigned Long Integer(number=w3095) -> (unsigned 32bit integer=w3094:u32[])
    n2075 = Join Numbers(hi=w3097, lo=w3096) -> ((hi.lo)=w3093:u32[])
    n2076 = Equal?(x=w3340, y=1.0) -> (x = y?=w3338:bool)
    n2077 = Join Numbers(hi=w3094, lo=w3093) -> ((hi.lo)=w3087:u64[])
    n2078 = call "IR AOM word to freq - vec.vi"("Frequency Word In (double vec)"=w3087) -> ("Frequency Out"=w3134:dbl[])
    n2079 = case "Alert buffer overflow" shown="True" w3338 {
      frame False {
      }
      frame True {
        n2080 = call <vilib>:"Beep.vi"() -> ()  [unwired: 3 in, 9 out]
        "Overflow (data lost)" <- TRUE ("Overflow (data lost)")
      }
    }
    n2081 = Decimate 1D Array(w3134) -> (w3133:dbl[], w3132:dbl[])
    n2082 = Build Array(w3133, w3132) -> (w3131:dbl[][])
    n2083 = local read "Trap Sets"() -> (w3209:u32)
    n2084 = case "Deinterlace trap data, average down PSD" shown="2" w3209 {
      tunnel: w3099 -> [w3872 w3937]
      tunnel: [w3869 w3934] -> w3202
      tunnel: [w3872 w3936] -> w3090
      tunnel: "Detector Type" -> [w3871 w3932]
      tunnel: [w3870 w3935] -> w3201
      tunnel: [w3868 w3933] -> w3315
      frame 1, Default {
        n2085 = Divide(x=w3872, y=3276.7) -> (x/y=w3873:dbl[])
        n2086 = Decimate 1D Array(w3873) -> (w3882:dbl[], w3881:dbl[], w3880:dbl[], w3879:dbl[], w3878:dbl[], w3877:dbl[], w3876:dbl[], w3875:dbl[])
        n2087 = case shown="\"IR-QPD + PSD + FB-QPD position\"" w3871 {
          tunnel: w3882 -> [w3906 w3931]
          tunnel: w3881 -> [w3905 w3930]
          tunnel: w3880 -> [w3890 w3908]
          tunnel: w3879 -> [w3891 w3918]
          tunnel: w3878 -> [w3904 w3929]
          tunnel: w3877 -> [w3903 w3928]
          tunnel: w3876 -> [w3887 w3909]
          tunnel: w3875 -> [w3886 w3907]
          tunnel: [w3885 w3915] -> w3870
          tunnel: [w3884 w3914] -> w3869
          tunnel: [w3883 w3913] -> w3868
          frame "IR-QPD + PSD + FB-QPD", Default {
            w3883 = 0  # Channel pattern
            n2088 = Divide(x=w3906, y=w3891) -> (x/y=w3893:dbl[])
            n2089 = Divide(x=w3905, y=w3891) -> (x/y=w3892:dbl[])
            n2090 = Divide(x=w3904, y=w3887) -> (x/y=w3889:dbl[])
            n2091 = Divide(x=w3903, y=w3886) -> (x/y=w3888:dbl[])
            n2092 = Build Array(w3893, w3892, w3891, w3890, w3889, w3888, w3887, w3886) -> (w3884:dbl[][])
            n2093 = Bundle("T1 Y", "T1 X", "T1 Sum", "FB Sum", "PSD Y", "PSD X", "PSD Y Sum", "PSD X Sum") -> (w3902:T40)  [unwired: 1 out]
            n2094 = Cluster To Array(cluster=w3902) -> (array=w3885:string[])
          }
          frame "IR-QPD + PSD + FB-QPD position" {
            w3913 = 3  # Channel pattern
            n2095 = Negate(x=w3909) -> (-x=w3910:dbl[])
            n2096 = Divide(x=w3931, y=w3918) -> (x/y=w3920:dbl[])
            n2097 = Divide(x=w3930, y=w3918) -> (x/y=w3919:dbl[])
            n2098 = Divide(x=w3929, y=w3909) -> (x/y=w3917:dbl[])
            n2099 = Divide(x=w3928, y=w3910) -> (x/y=w3916:dbl[])
            n2100 = Build Array(w3920, w3919, w3918, w3907, w3908, w3917, w3916, w3909) -> (w3914:dbl[][])
            n2101 = Bundle("T1 Y", "T1 X", "T1 Sum", "FB X", "FB Sum", "PSD Y", "PSD X", "PSD Y Sum") -> (w3927:T40)  [unwired: 1 out]
            n2102 = Cluster To Array(cluster=w3927) -> (array=w3915:string[])
          }
        }
      }
      frame 2 {
        n2103 = case shown="\"IR-QPD + PSD + FB-QPD X position\"" w3932 {
          tunnel: w3937 -> [w3999 w4066 w4137]
          tunnel: [w3938 w4057 w4068] -> w3936
          tunnel: [w3965 w4048 w4115] -> w3935
          tunnel: [w3964 w4011 w4082] -> w3934
          tunnel: [w3958 w4046 w4113] -> w3933
          frame "IR-QPD + PSD + FB-QPD", Default {
            w3958 = 1  # Channel pattern
            # "time average x2 the 4th signal and the 4 psd signals (detection laser)"
            # "deinterlace 3 signals from qpd"
            n2104 = Decimate 1D Array(w3999) -> (w3998:i16[], w3997:i16[], w3963:i16[], w3996:i16[], w3986:i16[], w3984:i16[], w3983:i16[], w3981:i16[])
            n2105 = Decimate 1D Array(w3963) -> (w3962:i16[], w3961:i16[])
            n2106 = Decimate 1D Array(w3998) -> (w3995:i16[], w3967:i16[])
            n2107 = Decimate 1D Array(w3997) -> (w3994:i16[], w3992:i16[])
            n2108 = Decimate 1D Array(w3996) -> (w3993:i16[], w3991:i16[])
            n2109 = call "downsample 1D array - double.vi"("Ave N"=2.0, "Array In"=w3986) -> ("Array Out"=w3985:dbl[])  [unwired: 1 out]
            n2110 = call "downsample 1D array - double.vi"("Ave N"=2.0, "Array In"=w3984) -> ("Array Out"=w3966:dbl[])  [unwired: 1 out]
            n2111 = call "downsample 1D array - double.vi"("Ave N"=2.0, "Array In"=w3983) -> ("Array Out"=w3982:dbl[])  [unwired: 1 out]
            n2112 = call "downsample 1D array - double.vi"("Ave N"=2.0, "Array In"=w3981) -> ("Array Out"=w3980:dbl[])  [unwired: 1 out]
            n2113 = Interleave 1D Arrays(w3995, w3994, w3993, w3967, w3992, w3991, w3962, w3961, w3985, w3966, w3982, w3980) -> (w3979:dbl[])
            n2114 = Divide(x=w3979, y=3276.7) -> (x/y=w3978:dbl[])
            n2115 = Decimate 1D Array(w3978) -> (w3977:dbl[], w3976:dbl[], w3975:dbl[], w3974:dbl[], w3973:dbl[], w3972:dbl[], w3960:dbl[], w3959:dbl[], w3971:dbl[], w3970:dbl[], w3969:dbl[], w3968:dbl[])
            n2116 = Divide(x=w3977, y=w3975) -> (x/y=w3945:dbl[])
            n2117 = Divide(x=w3976, y=w3975) -> (x/y=w3944:dbl[])
            n2118 = Divide(x=w3974, y=w3972) -> (x/y=w3943:dbl[])
            n2119 = Divide(x=w3973, y=w3972) -> (x/y=w3942:dbl[])
            n2120 = Divide(x=w3971, y=w3969) -> (x/y=w3941:dbl[])
            n2121 = Divide(x=w3970, y=w3968) -> (x/y=w3940:dbl[])
            n2122 = Build Array(w3945, w3944, w3975, w3943, w3942, w3972, w3960, w3959, w3941, w3940, w3969, w3968) -> (w3964:dbl[][])
            n2123 = Bundle("T1 Y", "T1 X", "T1 Sum", "T2 Y", "T2 X", "T2 Sum", "T1 FB Sum", "T2 FB Sum", "PSD Y", "PSD X", "PSD Y Sum", "PSD X Sum") -> (w3946:T41)  [unwired: 1 out]
            n2124 = To Word Integer(number=w3979) -> (16bit integer=w3938:i16[])
            n2125 = Cluster To Array(cluster=w3946) -> (array=w3965:string[])
          }
          frame "IR-QPD + PSD + FB-QPD X position" {
            w4046 = 2  # Channel pattern
            # "time average x2 the 3 psd signals (detection laser)"
            # "deinterlace 3 signals from qpds"
            n2126 = Decimate 1D Array(w4066) -> (w4065:i16[], w4064:i16[], w4047:i16[], w4063:i16[], w4009:i16[], w4006:i16[], w4003:i16[], w4034:i16[])
            n2127 = Decimate 1D Array(w4047) -> (w4032:i16[], w4030:i16[])
            n2128 = Decimate 1D Array(w4065) -> (w4062:i16[], w4049:i16[])
            n2129 = Decimate 1D Array(w4064) -> (w4061:i16[], w4059:i16[])
            n2130 = Decimate 1D Array(w4063) -> (w4060:i16[], w4058:i16[])
            n2131 = Decimate 1D Array(w4034) -> (w4033:i16[], w4031:i16[])
            n2132 = call "downsample 1D array - I16.vi"("Ave N"=2.0, "Array In"=w4009) -> ("Array Out"=w4007:i16[])  [unwired: 1 in]
            n2133 = call "downsample 1D array - I16.vi"("Ave N"=2.0, "Array In"=w4003) -> ("Array Out"=w4001:i16[])  [unwired: 1 in]
            n2134 = call "downsample 1D array - I16.vi"("Ave N"=2.0, "Array In"=w4006) -> ("Array Out"=w4004:i16[])  [unwired: 1 in]
            n2135 = Interleave 1D Arrays(w4062, w4061, w4060, w4049, w4059, w4058, w4033, w4032, w4031, w4030, w4007, w4004, w4001) -> (w4057:i16[])
            n2136 = Divide(x=w4057, y=3276.7) -> (x/y=w4056:dbl[])
            n2137 = Decimate 1D Array(w4056) -> (w4055:dbl[], w4054:dbl[], w4053:dbl[], w4052:dbl[], w4051:dbl[], w4050:dbl[], w4022:dbl[], w4020:dbl[], w4019:dbl[], w4017:dbl[], w4016:dbl[], w4015:dbl[], w4012:dbl[])
            n2138 = Negate(x=w4012) -> (-x=w4010:dbl[])
            n2139 = Divide(x=w4016, y=w4012) -> (x/y=w4014:dbl[])
            n2140 = Divide(x=w4015, y=w4010) -> (x/y=w4013:dbl[])
            n2141 = Divide(x=w4055, y=w4053) -> (x/y=w4038:dbl[])
            n2142 = Divide(x=w4054, y=w4053) -> (x/y=w4037:dbl[])
            n2143 = Divide(x=w4052, y=w4050) -> (x/y=w4036:dbl[])
            n2144 = Divide(x=w4051, y=w4050) -> (x/y=w4035:dbl[])
            n2145 = Divide(x=w4022, y=w4020) -> (x/y=w4021:dbl[])
            n2146 = Divide(x=w4019, y=w4017) -> (x/y=w4018:dbl[])
            n2147 = Build Array(w4038, w4037, w4053, w4036, w4035, w4050, w4021, w4020, w4018, w4017, w4014, w4013, w4012) -> (w4011:dbl[][])
            n2148 = Bundle("T1 Y", "T1 X", "T1 Sum", "T2 Y", "T2 X", "T2 Sum", "T1 FB X", "T1 FB Sum", "T2 FB X", "T2 FB Sum", "PSD Y", "PSD X", "PSD Y Sum") -> (w4039:T42)  [unwired: 1 out]
            n2149 = Cluster To Array(cluster=w4039) -> (array=w4048:string[])
          }
          frame "IR-QPD + PSD + FB-QPD XY positions" {
            w4113 = 4  # Channel pattern
            # "time average x2 the 3 psd signals (detection laser)"
            # "deinterlace 3 signals from qpds"
            n2150 = Decimate 1D Array(w4137) -> (w4136:i16[], w4135:i16[], w4114:i16[], w4134:i16[], w4080:i16[], w4126:i16[], w4125:i16[], w4102:i16[])
            n2151 = Decimate 1D Array "Feedback Sum"(w4114) -> (w4098:i16[], w4096:i16[])
            n2152 = Decimate 1D Array "QPD Y"(w4136) -> (w4133:i16[], w4116:i16[])
            n2153 = Decimate 1D Array "QPD X"(w4135) -> (w4132:i16[], w4130:i16[])
            n2154 = Decimate 1D Array "Feedback Y"(w4080) -> (w4079:i16[], w4078:i16[])
            n2155 = Decimate 1D Array "QPD Sum"(w4134) -> (w4131:i16[], w4129:i16[])
            n2156 = Decimate 1D Array "Feedback X"(w4102) -> (w4099:i16[], w4097:i16[])
            n2157 = call "downsample 1D array - double.vi"("Ave N"=2.0, "Array In"=w4126) -> ("Array Out"=w4101:dbl[])  [unwired: 1 out]
            n2158 = call "downsample 1D array - double.vi"("Ave N"=2.0, "Array In"=w4125) -> ("Array Out"=w4100:dbl[])  [unwired: 1 out]
            n2159 = Interleave 1D Arrays(w4133, w4132, w4131, w4116, w4130, w4129, w4079, w4099, w4098, w4078, w4097, w4096, w4101, w4100) -> (w4124:dbl[])
            n2160 = Divide(x=w4124, y=3276.7) -> (x/y=w4123:dbl[])
            n2161 = Decimate 1D Array(w4123) -> (w4122:dbl[], w4121:dbl[], w4120:dbl[], w4119:dbl[], w4118:dbl[], w4117:dbl[], w4075:dbl[], w4089:dbl[], w4073:dbl[], w4074:dbl[], w4087:dbl[], w4071:dbl[], w4085:dbl[], w4083:dbl[])
            n2162 = Negate(x=w4083) -> (-x=w4081:dbl[])
            n2163 = Divide(x=w4085, y=w4081) -> (x/y=w4084:dbl[])
            n2164 = Divide(x=w4074, y=w4071) -> (x/y=w4070:dbl[])
            n2165 = Divide(x=w4075, y=w4073) -> (x/y=w4072:dbl[])
            n2166 = Divide(x=w4122, y=w4120) -> (x/y=w4106:dbl[])
            n2167 = Divide(x=w4121, y=w4120) -> (x/y=w4105:dbl[])
            n2168 = Divide(x=w4119, y=w4117) -> (x/y=w4104:dbl[])
            n2169 = Divide(x=w4118, y=w4117) -> (x/y=w4103:dbl[])
            n2170 = Divide(x=w4089, y=w4073) -> (x/y=w4088:dbl[])
            n2171 = Divide(x=w4087, y=w4071) -> (x/y=w4086:dbl[])
            n2172 = Build Array(w4106, w4105, w4120, w4104, w4103, w4117, w4072, w4088, w4073, w4070, w4086, w4071, w4084, w4083) -> (w4082:dbl[][])
            n2173 = Bundle("T1 Y", "T1 X", "T1 Sum", "T2 Y", "T2 X", "T2 Sum", "T1 FB Y", "T1 FB X", "T1 FB Sum", "T2 FB Y", "T2 FB X", "T2 FB Sum", "PSD X", "PSD Y Sum") -> (w4069:T43)  [unwired: 1 out]
            n2174 = To Word Integer(number=w4124) -> (16bit integer=w4068:i16[])
            n2175 = Cluster To Array(cluster=w4069) -> (array=w4115:string[])
          }
        }
      }
    }
    "AI labels" <- w3201
    n2176 = Decimate 1D Array(w3175) -> (w3199:u32[], w3143:u32[])
    n2177 = local read "DMA Update Period (s)"() -> (w3211:dbl)
    n2178 = Build Array(w3199, w3143) -> (w3277:u32[][])
    n2179 = local read "Data Period (s)"() -> (w3049:dbl)
    n2180 = local read "BD 1 Frequency 2 (MHz)"() -> (w3082:dbl)
    n2181 = local read "BD 1 Frequency 1 (MHz)"() -> (w3083:dbl)
    n2182 = Decimate 1D Array(w3090) -> (w3114:i16[], w3113:i16[], w3111:i16[], w3110:i16[])  [unwired: 9 out]
    n2183 = To Double Precision Float(number=w3277) -> (double precision float=w3278:dbl[][])
    n2184 = local read "APD Integration Time (s)"() -> (w3156:dbl)
    n2185 = Multiply(x=w3049, y="Trap Pos. Disp. Downsample") -> (x*y=w3047:dbl)
    n2186 = Divide(x=w3114, y=w3113) -> (x/y=w3115:dbl[])
    n2187 = Divide(x=w3111, y=w3110) -> (x/y=w3112:dbl[])
    n2188 = feedback #6(0.0) -> (w3128:dbl)
    n2189 = Add(x=w3211, y=w3128) -> (x+y=w3317:dbl)
    n2190 = feedback-in #6(w3317) -> ()
    n2191 = local read "AOM X Cal (nm/MHz)"() -> (w3080:dbl)
    n2192 = To Time Stamp(1:w3128) -> (0:w3127:timestamp)
    n2193 = Split 1D Array(array=w3115, index="N El. to Ave.") -> (second subarray=w3118:dbl[])  [unwired: 1 out]
    n2194 = Split 1D Array(array=w3112, index="N El. to Ave.") -> (second subarray=w3117:dbl[])  [unwired: 1 out]
    n2195 = Multiply(x=w3049, y="Trap Disp. Downsample") -> (x*y=w3129:dbl)
    "Display Period (s)" <- w3129
    n2196 = for "Trap AI" {
      tunnel: [w3867] -> w3311 mode=indexing
      tunnel: w3127 -> [w3857]
      tunnel: "Trap Disp. Downsample" -> [w3865]
      tunnel: w3202 -> [w3863] mode=indexing
      tunnel: w3049 -> [w3862]
      tunnel: w3201 -> [w3861] mode=indexing
      tunnel: w3126 -> [w3860]
      tunnel: [w3859] -> w3167 mode=indexing
      tunnel: w3129 -> [w3858]
      workers-P: _ -> [_]
      n2197 = Bundle By Name("Y"=w3863, "dt"=w3862) -> (w3864:waveform(dbl))  [unwired: 1 out]
      n2198 = Set Waveform Attribute(5:w3861, 6:w3860, 7:w3864) -> (3:w3859:waveform(dbl))  [unwired: 1 in, 2 out]
      n2199 = call "downsample 1D array - double.vi"("Ave N"=w3865, "Array In"=w3863) -> ("Array Out"=w3866:dbl[])  [unwired: 1 out]
      n2200 = Bundle By Name(cluster=w3859, "t0"=w3857, "Y"=w3866, "dt"=w3858) -> (w3867:waveform(dbl))
    }
    n2201 = Bundle("BD 1 Frequency 1 (MHz)"=w3083, "BD 1 Frequency 2 (MHz)"=w3082) -> (w3084:T44)  [unwired: 1 out]
    n2202 = call <vilib>:"Mean.vi"("X"=w3117) -> ("mean"=w3105:dbl)  [unwired: 1 out]
    n2203 = call <vilib>:"Mean.vi"("X"=w3118) -> ("mean"=w3106:dbl)  [unwired: 1 out]
    n2204 = Reciprocal(x=w3129) -> (1/x=→"Trap Disp. Freq. (Hz)":dbl)
    n2205 = Cluster To Array(cluster=w3084) -> (array=w3081:dbl[])
    n2206 = local read "Trap X AI1 (DMA)"() -> (w3116:T13)
